vi "Test Configure.vi"(0 "Template Tx Test in":refnum<class "niDTS WLAN Tx Test.lvclass">, 11 "error in (no error)":errorcluster) -> (4 "Template Tx Test out":refnum<class "niDTS WLAN Tx Test.lvclass">, 15 "error out":errorcluster)   [LabVIEW 2015, in "niDTS WLAN.lvlib" / "niDTS WLAN Tx Test.lvclass"]
uses:
  niDTS WLAN Tx Test.lvclass
  niDTS WLAN Tx Test.lvclass/niDTS WLAN Tx Test.ctl
  RiviInstDriver/InstDriver/Objects/InstDriver.lvclass/InstDriver.ctl
  RiviInstDriver/InstDriver/Objects/Read VISA resource.vi
  TestStand/Station/Objects/SystemTechnologyCatalog/niDTS SystemTechnologyCatalog.lvclass
  TestStand/Station/Objects/SystemDut/niDTS SystemDut.lvclass
  Framework/Dut/Objects/BASE_class/niDTS Dut.lvclass
  Instrument/INSTR TX/niDTS WLAN INSTR TX.lvclass
  Dut/Objects/BASE_class/niDTS WLAN Dut.lvclass
  niDTS WLAN.lvlib
  Framework/niDTS Framework.lvlib
  TestStand/niDTS TestStand.lvlib
  RiviInstDriver/niRfsaWlan/Objects/niRfsaWlan.lvclass
  RiviInstDriver/InstDriver/Objects/InstDriver.lvclass
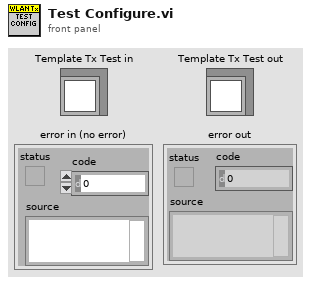
[diagram p1: front panel]
types:
  T1 = typedef "niDTS Framework.lvlib/niDTS Dut INC Handle.ctl" = refnum<data-value>
  T2 = typedef "niDTS WLAN.lvlib/niDTS WLAN Tx Test INC Parameters.ctl" = cluster{"Standard":T3, "DSSS Data Rate (Mbps)":T4, "OFDM Data Rate (Mbps)":T5, "MCS Index":i32, "N spatial streams":i32, "Chains":bool[], "BandWidth (Hz)":T6, "Channel":i32, "Gard Interval":T7, "FEC Coding":T8, "Dut Tx Power":dbl, "16 symbols":bool, "payload length bytes":i32, "idle interval":dbl, "External Attenuation":dbl[], "Acquisition Parameters ":T9, "TXP Measurement Parameters":T10, "ModAcc Measurement Paramaters":T11, "ModAcc DSSS Paramaters":T12, "SEM Measurement Parameters":T14, "OBW Measurement Parameters":T15, "DSSS Power Ramp":T16, "Enable Traces":bool}
  T3 = typedef "niDTS WLAN.lvlib/niDTS WLAN INC Standard.ctl" = enum16{"802.11 b DSSS", "802.11 a/g OFDM", "802.11 n HT", "802.11 ac VHT"}
  T4 = typedef "niDTS WLAN.lvlib/niDTS WLAN INC DSSS Data Rate.ctl" = enum16{"1", "2", "5.5", "11"}
  T5 = typedef "niDTS WLAN.lvlib/niDTS WLAN INC OFDM Data Rate.ctl" = enum16{"6", "9", "12", "18", "24", "36", "48", "54"}
  T6 = typedef "niDTS WLAN.lvlib/niDTS WLAN INC CH BW.ctl" = enum16{"20 MHz", "40 MHz", "80 MHz", "160 MHz"}
  T7 = typedef "niDTS WLAN.lvlib/niDTS WLAN INC GI.ctl" = enum16{"LONG", "SHORT"}
  T8 = typedef "niDTS WLAN.lvlib/niDTS WLAN INC FEC Coding.ctl" = enum16{"BCC", "LDPC"}
  T9 = typedef "niDTS WLAN.lvlib/niDTS WLAN DUT INC Acquisition Parameters.ctl" = cluster{"Acquisition Length Mode":enum16{"AUTO", "MANUAL"}, "Acquisition Length (s)":dbl, "Auto Level":bool}
  T10 = typedef "niDTS WLAN.lvlib/niDTS WLAN INC TXP Measurement Parameters.ctl" = cluster{"TXP Power Enable":bool, "TXP Averages":i32}
  T11 = typedef "niDTS WLAN.lvlib/niDTS WLAN INC ModAcc Measurement Parameters.ctl" = cluster{"ModAcc Enable":bool, "Header Detection":enum16{"MANUAL", "FIRST", "ALL"}, "Averages":i32, "Amplitude Tracking":bool, "Channel Tracking":bool, "Time Tracking":bool, "Phase Tracking":enum16{"NONE", "STANDARD", "CSF", "INSTANT"}, "Clock Offset Est":bool, "Impairments Est":bool, "CFO Estimation":enum16{"PAMBLE", "PDATA"}}
  T12 = typedef "niDTS WLAN.lvlib/niDTS WLAN INC DSSS ModAcc Measurement Parameters.ctl" = cluster{"DC Offset Compensation":bool, "Equalization":bool, "Phase Tracking":bool, "Chip Start Location":i16, "Max Chips Used":i16, "Pulse Shaping FilterType":T13, "Pulse Shaping Filter Coefficient":dbl}
  T13 = typedef "niDTS WLAN.lvlib/niDTS WLAN INC Pulse Shaping Filter Type.ctl" = enum16{"NONE", "RCOSINE", "RRCOSINE", "GAUSSIAN"}
  T14 = typedef "niDTS WLAN.lvlib/niDTS WLAN INC SEM Measurement Parameters.ctl" = cluster{"SEM Enable":bool, "SEM Averages":i32, "Auto Span Enable":bool, "Frequency Span (Hz)":dbl, "Measurement Type":enum16{"Standard", "Legacy", "Custom"}, "Mask Frequencies (Hz)":dbl[], "Mask Power Offsets (dB)":dbl[]}
  T15 = typedef "niDTS WLAN.lvlib/niDTS WLAN INC OBW Measurement Parameters.ctl" = cluster{"OBW Enable":bool, "OBW Averages":i32}
  T16 = typedef "niDTS WLAN.lvlib/niDTS WLAN INC DSSS Power Ramp Parameters.ctl" = cluster{"Power Ramp Enable":bool, "Averages":i32, "Thresholds":cluster{"Up Low (%)":dbl, "Down Low (%)":dbl, "Up High (%)":dbl, "Down High (%)":dbl}}
  T17 = typedef "InstDriver.lvclass/niInstDriver INC Handle.ctl" = refnum<data-value>
  T18 = typedef "niDTS WLAN.lvlib/niDTS WLAN DUT INC Parameters.ctl" = cluster{"WLAN Type":T19, "Bandwidth (Hz)":T6, "Channel":i32, "Guard Interval":T7, "FEC Coding":T8, "Power (dBm)":dbl, "Payload Length (bytes)":i32, "16 Symbols":bool, "Chains":bool[]}
  T19 = typedef "niDTS WLAN.lvlib/niDTS WLAN INC Type.ctl" = enum16{"b - 1 Mbps", "b - 2 Mbps", "b - 5.5 Mbps", "b - 11 Mbps", "ag - 6 Mbps", "ag - 9 Mbps", "ag - 12 Mbps", "ag - 18 Mbps", "ag - 24 Mbps", "ag - 36 Mbps", "ag - 48 Mbps", "ag - 54 Mbps", "n - MCS0", "n - MCS1", "n - MCS2", "n - MCS3", "n - MCS4", "n - MCS5", "n - MCS6", "n - MCS7", "n - MCS8", "n - MCS9", "n - MCS10", "n - MCS11", "n - MCS12", "n - MCS13", "n - MCS14", "n - MCS15", "n - MCS16", "n - MCS17", "n - MCS18", "n - MCS19", "n - MCS20", "n - MCS21", "n - MCS22", "n - MCS23", "n - MCS24", "n - MCS25", "n - MCS26", "n - MCS27", "n - MCS28", "n - MCS29", "n - MCS30", "n - MCS31", "ac - MCS0 -1", "ac - MCS1 -1", "ac - MCS2 -1", "ac - MCS3 -1", "ac - MCS4 -1", "ac - MCS5 -1", "ac - MCS6 -1", "ac - MCS7 -1", "ac - MCS8 -1", "ac - MCS9 -1", "ac - MCS0 -2", "ac - MCS1 -2", "ac - MCS2 -2", "ac - MCS3 -2", "ac - MCS4 -2", "ac - MCS5 -2", "ac - MCS6 -2", "ac - MCS7 -2", "ac - MCS8 -2", "ac - MCS9 -2", "ac - MCS0 -3", "ac - MCS1 -3", "ac - MCS2 -3", "ac - MCS3 -3", "ac - MCS4 -3", "ac - MCS5 -3", "ac - MCS6 -3", "ac - MCS7 -3", "ac - MCS8 -3", "ac - MCS9 -3", "ac - MCS0 -4", "ac - MCS1 -4", "ac - MCS2 -4", "ac - MCS3 -4", "ac - MCS4 -4", "ac - MCS5 -4", "ac - MCS6 -4", "ac - MCS7 -4", "ac - MCS8 -4", "ac - MCS9 -4"}
  T20 = typedef "niDTS WLAN.lvlib/niDTS WLAN Dut INC Handle.ctl" = refnum<data-value>
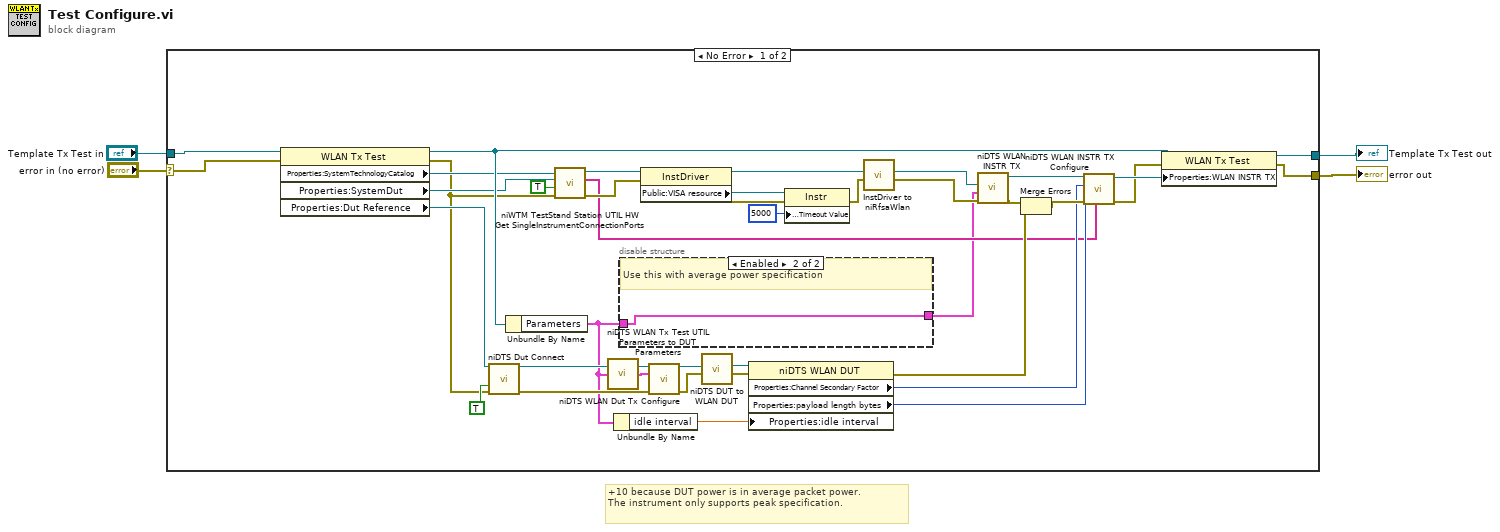
[diagram p0: block diagram]
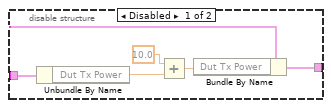
[diagram p2: hidden frame]
diagram:
  # "+10 because DUT power is in average packet power.\nThe instrument only supports peak specification."
  n1 = case shown="No Error" "error in (no error)" {
    selector: "error in (no error)" -> [w42 w51]
    tunnel: [w40 w51] -> w2
    tunnel: [w41 w50] -> w3
    tunnel: "Template Tx Test in" -> [w43 w50]
    frame No Error {
      n2 = property class="WLAN Tx Test"(reference=w43, error in=w42) -> (reference out=w21:refnum<class "niDTS WLAN Tx Test.lvclass">, error out=w14:errorcluster, "Properties:SystemTechnologyCatalog"=w17:refnum<class "niDTS SystemTechnologyCatalog.lvclass">, "Properties:SystemDut"=w16:refnum<class "niDTS SystemDut.lvclass">, "Properties:Dut Reference"=w36:T1)
      n3 = call "niDTS Dut Connect.vi"("Dut Handle"=w36, "Auto Interface"=TRUE, "error in (no error)"=w14) -> ("Dut Handle out"=w37:T1, "error out"=w35:errorcluster)  [unwired: 11 in]
      n4 = Unbundle By Name(w21) -> ("Parameters"=w6:T2)
      n5 = call "niWTM TestStand Station UTIL HW Get SingleInstrumentConnectionPorts.vi"("error in (no error)"=w14, "TX Instrument"=TRUE, "SystemDut"=w16, "SystemTechnologyCatalog"=w17) -> ("error out"=w12:errorcluster, "Ports"=w7:string[], "InstDriver Handle"=w13:T17)  [unwired: 5 in]
      n6 = call "niDTS WLAN Tx Test UTIL Parameters to DUT Parameters.vi"("Parameters"=w6) -> ("TV Parameters(DataType)"=w39:T18)  [unwired: 14 in]
      n7 = Unbundle By Name(w6) -> ("idle interval"=w28:dbl)
      n8 = disable-structure shown="Enabled" {
        disable-tunnel: w6 -> [w46 w49]
        disable-tunnel: [w44 w49] -> w5
        frame Disabled {
          n9 = Unbundle By Name(w46) -> ("Dut Tx Power"=w48:dbl)
          n10 = Add(x=10.0, y=w48) -> (x+y=w45:dbl)
          n11 = Bundle By Name(cluster=w46, "Dut Tx Power"=w45) -> (w44:T2)
        }
        frame Enabled {
          # "Use this with average power specification"
        }
      }
      n12 = property class="InstDriver"(reference=w13, error in=w12) -> (reference out=w11:T17, error out=w27:errorcluster, "Public:VISA resource"=w33:refnum<visa-resource-name>)
      n13 = call "niDTS WLAN Dut Tx Configure.vi"("Dut Handle in"=w37, "niDTS WLAN DUT Parameters"=w39, "error in (no error)"=w35) -> ("Dut Handle"=w30:T1, "error out"=w29:errorcluster)  [unwired: 11 in]
      n14 = call "niDTS DUT to WLAN DUT.vi"("error in"=w29, "Dut Handle"=w30) -> ("error out"=w32:errorcluster, "WLAN Dut Handle"=w31:T20)  [unwired: 8 in]
      n15 = property class="niDTS WLAN DUT"(reference=w31, error in=w32, "Properties:idle interval"=w28) -> (error out=w18:errorcluster, "Properties:Channel Secondary Factor"=w23:i8, "Properties:payload length bytes"=w22:i32)  [unwired: 1 out]
      n16 = property class="Instr"(reference=w33, error in=w27, "General Settings:Timeout Value"=u32 5000) -> (error out=w8:errorcluster)  [unwired: 1 out]
      n17 = call "InstDriver to niRfsaWlan.vi"("error in (no error)"=w8, "InstDriver Handle in"=w11) -> ("error out"=w9:errorcluster, "InstDriver Handle out"=w10:refnum<data-value>)  [unwired: 8 in]
      n18 = call "niDTS WLAN INSTR TX.vi"("error in (no error)"=w9, "WLAN Tx Input Parameters"=w5, "RfsaWlan Handle"=w10) -> ("error out"=w25:errorcluster, "niDTS WLAN INSTR TX"=w26:refnum<class "niDTS WLAN INSTR TX.lvclass">)  [unwired: 7 in]
      n19 = Merge Errors(w25, w18) -> (w24:errorcluster)
      n20 = call-dynamic "niDTS WLAN INSTR TX Configure.vi"("Port Names"=w7, "error in (no error)"=w24, "Payload length bytes"=w22, "Channel Secondary Factor"=w23, "niDTS WLAN INSTR TX in"=w26) -> ("error out"=w19:errorcluster, "niDTS WLAN INSTR TX out"=w20:refnum<class "niDTS WLAN INSTR TX.lvclass">)  [unwired: 5 in]
      n21 = property class="WLAN Tx Test"(reference=w21, error in=w19, "Properties:WLAN INSTR TX"=w20) -> (reference out=w41:refnum<class "niDTS WLAN Tx Test.lvclass">, error out=w40:errorcluster)
    }
    frame Error {
    }
  }
  "error out" <- w2
  "Template Tx Test out" <- w3
